vi "DSPS_E36000.Set Output Voltage.vi"(6 "CurLim":dbl=1.0 caption="Current Limit(A)", 8 "error in":errorcluster, 9 "State":bool, 10 "Voltage":dbl, 11 "VISA Alias":refnum<visa-resource-name>) -> (0 "error out":errorcluster, 3 "VISA Alias Dup":refnum<visa-resource-name>)   [LabVIEW 2018]
uses:
  <vilib>/KATE/Time/Time Utils.lvlib
panel:
  out "Duration(s)":dbl
  out "Error":string
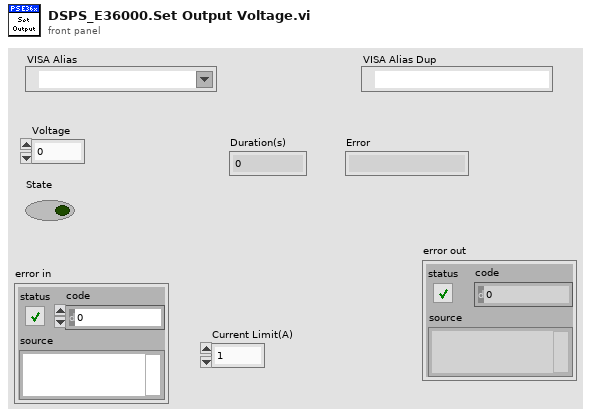
[diagram p1: front panel]
types:
  T1 = cluster{"State":bool, "CurLim":dbl, "Voltage":dbl}
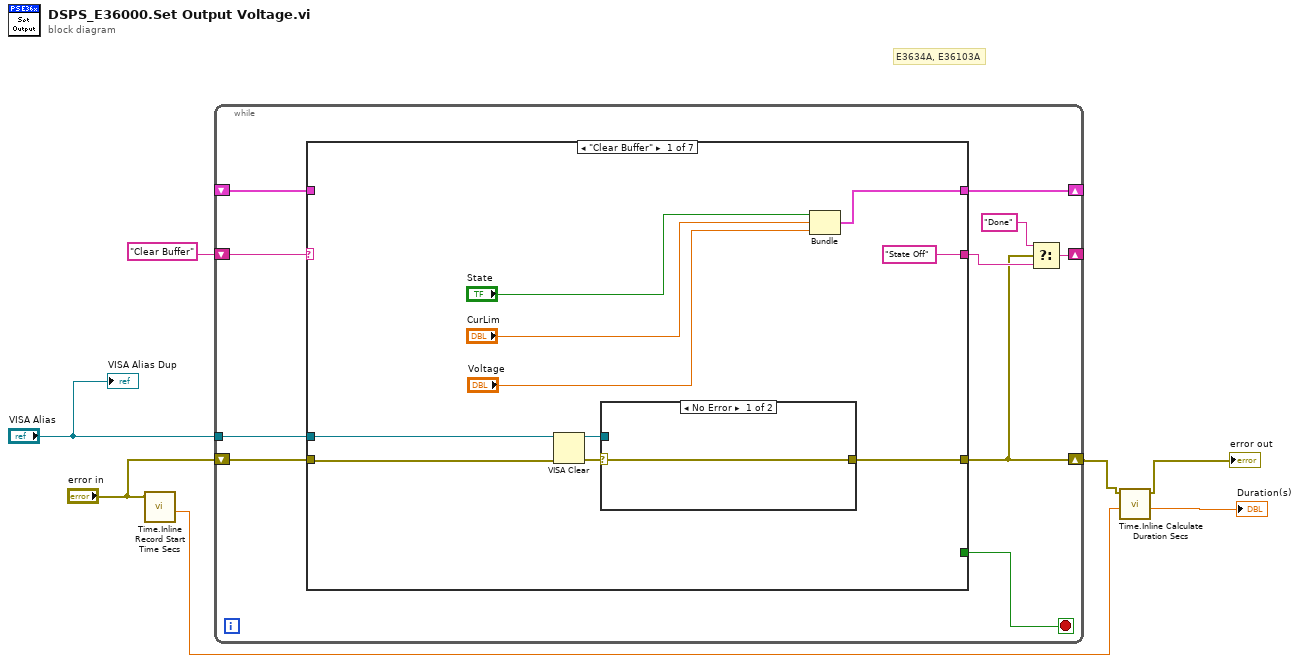
[diagram p0: block diagram]
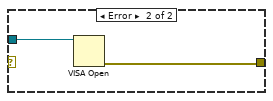
[diagram p2: hidden frame]
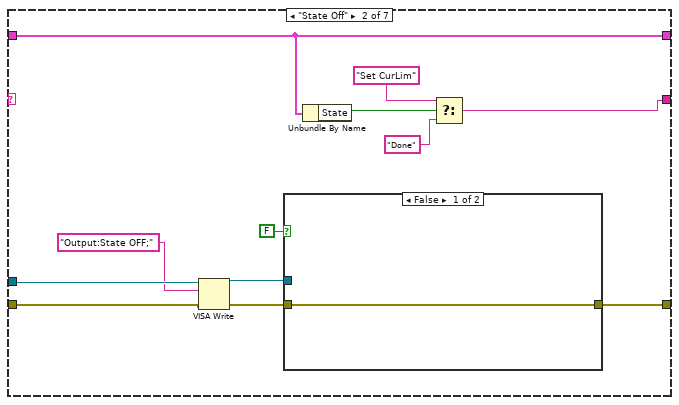
[diagram p3: hidden frame]
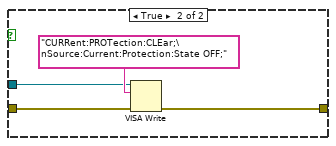
[diagram p4: hidden frame]
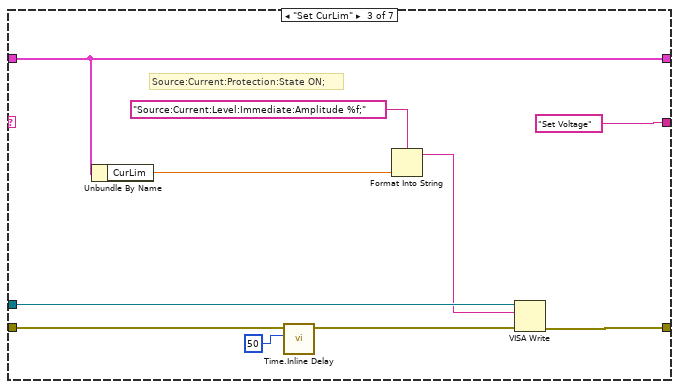
[diagram p5: hidden frame]
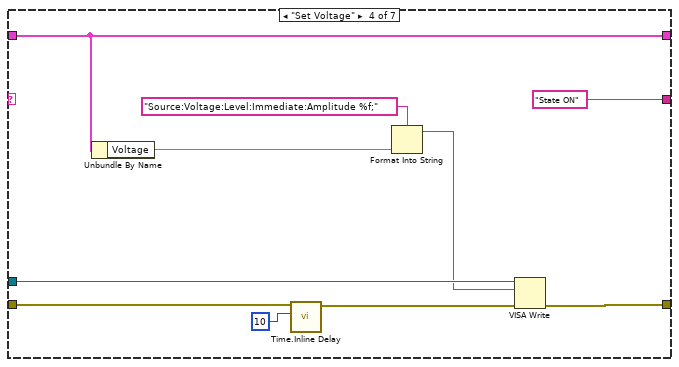
[diagram p6: hidden frame]
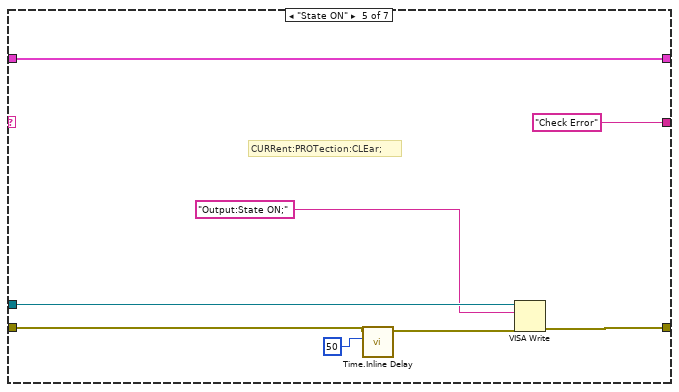
[diagram p7: hidden frame]
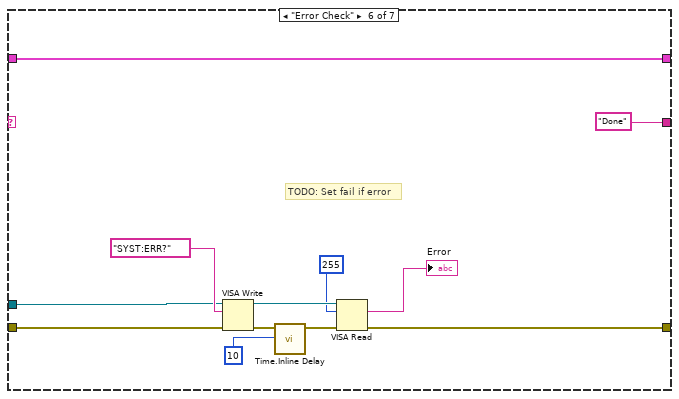
[diagram p8: hidden frame]
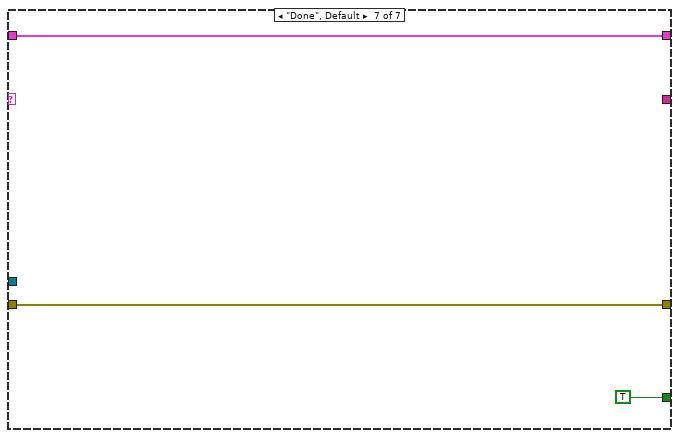
[diagram p9: hidden frame]
diagram:
  # "E3634A, E36103A"
  n1 = call <vilib>:"Time.Inline Record Start Time Secs.vi"("Error In Upper"="error in") -> ("Start(s)"=w3:dbl)  [unwired: 8 in, 2 out]
  n2 = while {
    shift-right: [w13] -> _
    shift-left: _ -> [w16]
    shift-right: [w10] -> _
    shift-left: "Clear Buffer" -> [w17]
    tunnel: "VISA Alias" -> [w15]
    shift-right: [w9] -> w4
    shift-left: "error in" -> [w14]
    stop <- w8 stop-if-true
    n3 = case shown="\"Clear Buffer\"" w17 {
      tunnel: w16 -> [_ w41 w55 w65 w73 w80 w89]
      tunnel: w15 -> [w22 w36 w57 w67 w75 w84 _]
      tunnel: w14 -> [w21 w34 w50 w59 w69 w82 w88]
      tunnel: [w18 w42 w56 w66 w74 w83 w88] -> w9
      tunnel: [w24 w41 w55 w65 w73 w80 w89] -> w13
      tunnel: ["State Off" w39 "Set Voltage" "State ON" "Check Error" "Done" _] -> w11
      tunnel: [_ _ _ _ _ _ TRUE] -> w8
      frame "Clear Buffer" {
        n4 = VISA Clear(VISA resource name=w22, error in (no error)=w21) -> (VISA resource name out=w19:refnum<visa-resource-name>, error out=w20:errorcluster)
        n5 = case shown="No Error" w20 {
          selector: w20 -> [w28 _]
          tunnel: w19 -> [_ w30]
          tunnel: [w28 w29] -> w18
          frame No Error {
          }
          frame Error {
            n6 = VISA Open(VISA resource name=w30) -> (error out=w29:errorcluster)  [unwired: 4 in, 1 out]
          }
        }
        n7 = Bundle("State"="State", "CurLim"="CurLim", "Voltage"="Voltage") -> (w24:T1)  [unwired: 1 in]
      }
      frame "State Off" {
        n8 = VISA Write(VISA resource name=w36, write buffer="Output:State OFF;", error in (no error)=w34) -> (VISA resource name out=w33:refnum<visa-resource-name>, error out=w32:errorcluster)  [unwired: 1 out]
        n9 = case shown="False" FALSE {
          tunnel: [w43 w46] -> w42
          tunnel: w33 -> [_ w45]
          tunnel: w32 -> [w43 w44]
          frame False {
          }
          frame True {
            n10 = VISA Write(VISA resource name=w45, write buffer="CURRent:PROTection:CLEar;\nSource:Current:Protection:State OFF;", error in (no error)=w44) -> (error out=w46:errorcluster)  [unwired: 2 out]
          }
        }
        n11 = Unbundle By Name(w41) -> ("State"=w40:bool)
        n12 = Select(t="Set CurLim", s=w40, f="Done") -> (s? t:f=w39:string)
      }
      frame "Set CurLim" {
        # "Source:Current:Protection:State ON;"
        n13 = Unbundle By Name(w55) -> ("CurLim"=w52:dbl)
        n14 = call <vilib>:"Time.Inline Delay.vi"("Wait(ms)"=u32 50, "error in top"=w50) -> ("error out top"=w49:errorcluster)  [unwired: 8 in, 1 out]
        n15 = Format Into String(format string="Source:Current:Level:Immediate:Amplitude %f;", w52) -> (resulting string=w51:string)  [unwired: 2 in, 1 out]
        n16 = VISA Write(VISA resource name=w57, write buffer=w51, error in (no error)=w49) -> (error out=w56:errorcluster)  [unwired: 2 out]
      }
      frame "Set Voltage" {
        n17 = Unbundle By Name(w65) -> ("Voltage"=w62:dbl)
        n18 = call <vilib>:"Time.Inline Delay.vi"("Wait(ms)"=u32 10, "error in top"=w59) -> ("error out top"=w58:errorcluster)  [unwired: 8 in, 1 out]
        n19 = Format Into String(format string="Source:Voltage:Level:Immediate:Amplitude %f;", w62) -> (resulting string=w61:string)  [unwired: 2 in, 1 out]
        n20 = VISA Write(VISA resource name=w67, write buffer=w61, error in (no error)=w58) -> (error out=w66:errorcluster)  [unwired: 2 out]
      }
      frame "State ON" {
        # "CURRent:PROTection:CLEar;"
        n21 = call <vilib>:"Time.Inline Delay.vi"("Wait(ms)"=u32 50, "error in top"=w69) -> ("error out top"=w68:errorcluster)  [unwired: 8 in, 1 out]
        n22 = VISA Write(VISA resource name=w75, write buffer="Output:State ON;", error in (no error)=w68) -> (error out=w74:errorcluster)  [unwired: 2 out]
      }
      frame "Error Check" {
        # "TODO: Set fail if error"
        n23 = VISA Write(VISA resource name=w84, write buffer="SYST:ERR?", error in (no error)=w82) -> (VISA resource name out=w87:refnum<visa-resource-name>, error out=w78:errorcluster)  [unwired: 1 out]
        n24 = call <vilib>:"Time.Inline Delay.vi"("Wait(ms)"=u32 10, "error in top"=w78) -> ("error out top"=w77:errorcluster)  [unwired: 8 in, 1 out]
        n25 = VISA Read(VISA resource name=w87, byte count=u32 255 ("byte count (0)"), error in (no error)=w77) -> (read buffer=→"Error":string, error out=w83:errorcluster)  [unwired: 2 out]
      }
      frame "Done", Default {
      }
    }
    n26 = Select(t="Done", s=w9, f=w11) -> (s? t:f=w10:string)
  }
  n27 = call <vilib>:"Time.Inline Calculate Duration Secs.vi"("Start(Sec)"=w3, "Error In Top"=w4) -> ("Duration(s)"=→"Duration(s)":dbl, "Error Out Top"=→"error out":errorcluster)  [unwired: 7 in, 1 out]
  "VISA Alias Dup" <- "VISA Alias"
